vi "Example After.vi"() -> ()   [LabVIEW 2019, in "LSS.lvlib"]
doc: "This example demonstrates how a user can save time developing user interfaces using LSS by showing how a simple application that uses property nodes to change style at runtime can be transitioned to using LSS. The \"Example Before.vi\" contains one way the code could have been written using arrays of property nodes. The \"Example After.vi\" is a functionally equivalent piece of code that uses LSS instead. Example After.vi uses no property nodes or manually created references to perform the exact same operations."
uses:
  LSS.lvlib
  SubVIs/Example SubVIs/Before SubVIs/Themes.ctl
panel:
  in  "CUSTOM":bool
  out "mode":T1
  in  "DIALOG":bool
  in  "NORMAL":bool
  in  "SMALL":bool
  in  "Slide 2":dbl(slide) scale=0.0..10.0
  out "Stat2":dbl
  out "Stat1":dbl
  out "Pressure":dbl
  out "Time":dbl
  in  "Slide":dbl(slide) scale=0.0..10.0
  in  "THEME2":bool
  in  "THEME1":bool
  in  "COMPANY":bool
  in  "SPACE":bool
  out "Mars":picture
  out "Map":picture
  out "SLS":picture
  out "Chart3":dbl(graph)
  out "Chart2":dbl(graph)
  out "Chart1":dbl(graph)
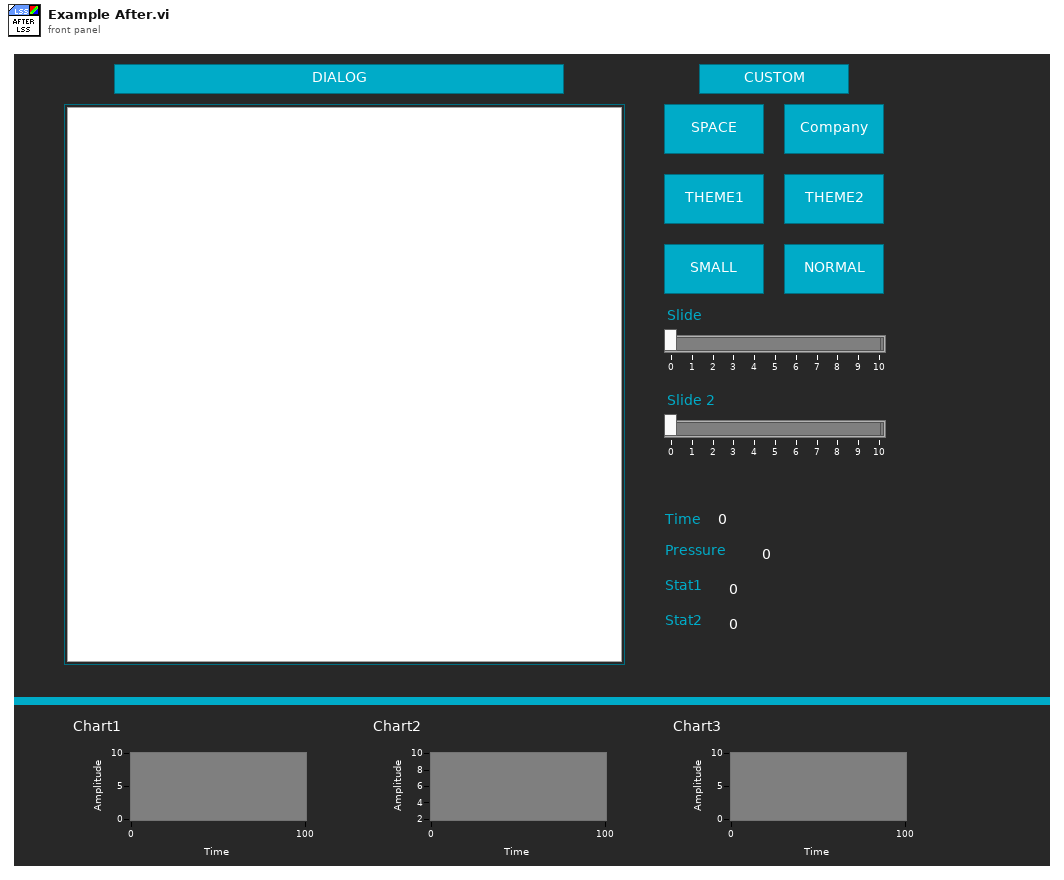
[diagram p1: front panel]
types:
  T1 = typedef "LSS.lvlib/Themes.ctl" = enum16{"SPACE", "COMPANY", "THEME1", "THEME2"}
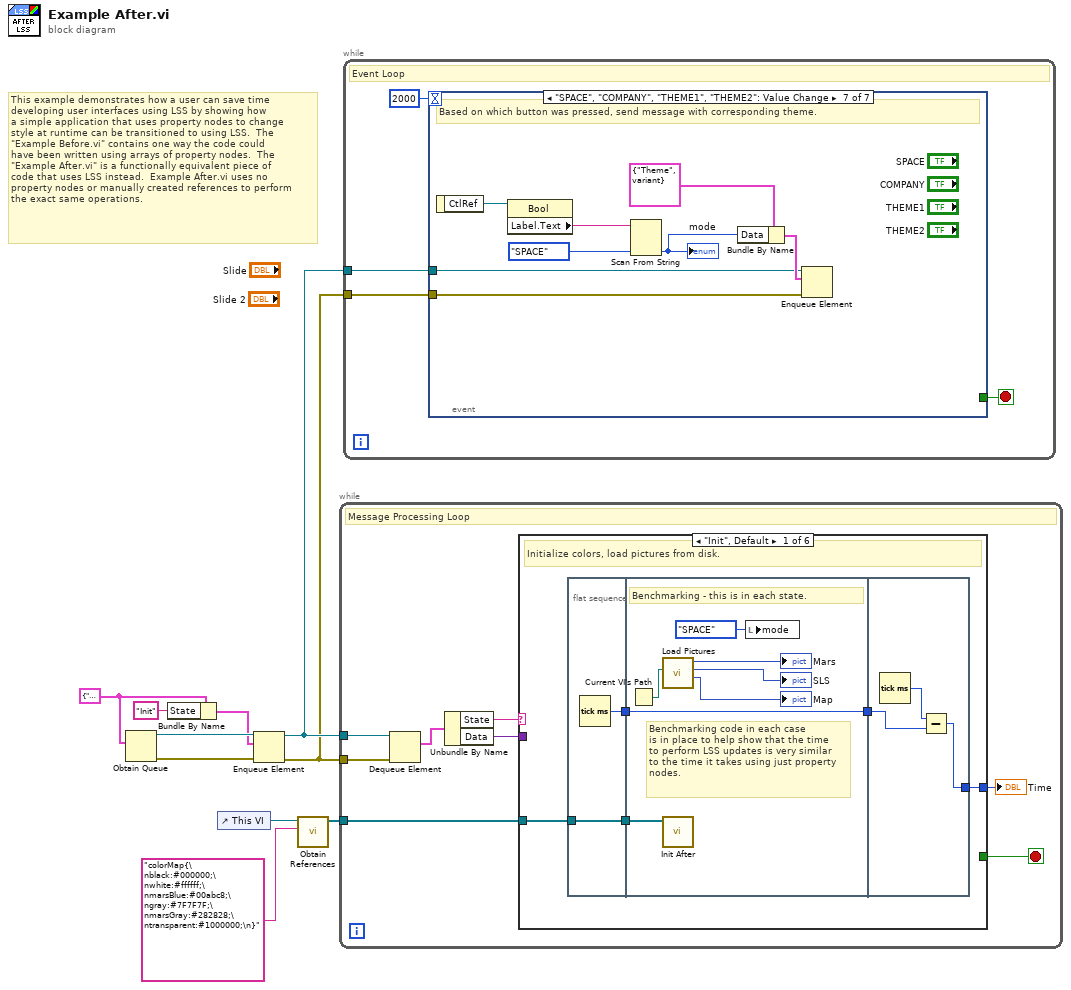
[diagram p0: block diagram]
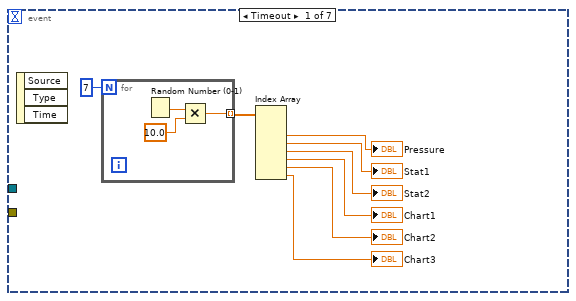
[diagram p2: hidden frame]
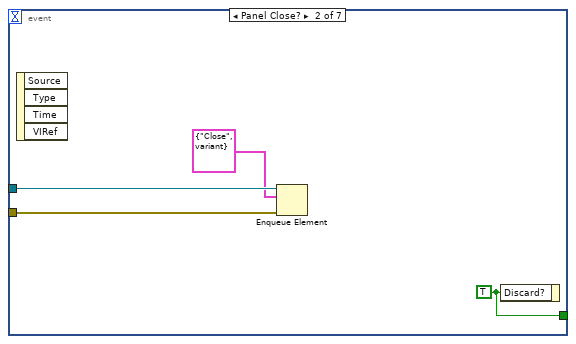
[diagram p3: hidden frame]
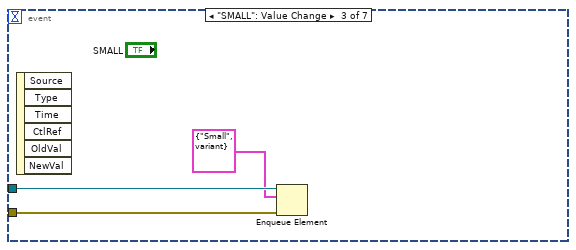
[diagram p4: hidden frame]
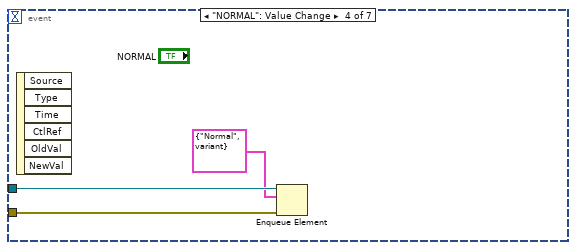
[diagram p5: hidden frame]
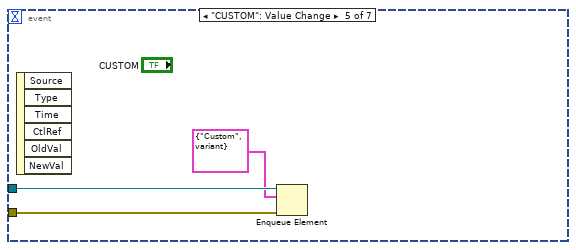
[diagram p6: hidden frame]
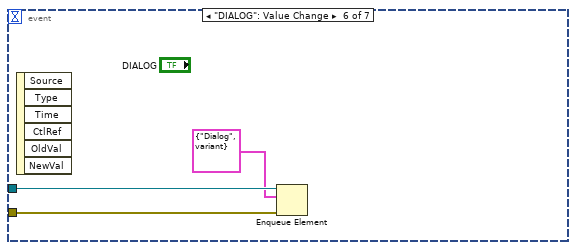
[diagram p7: hidden frame]
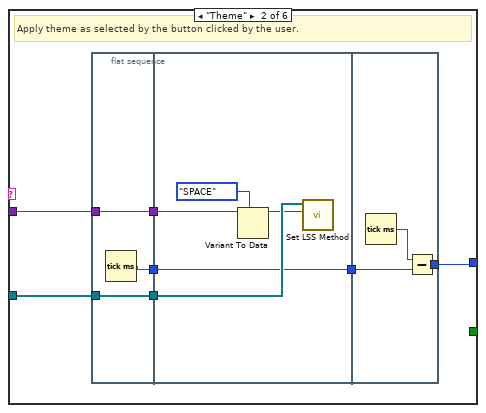
[diagram p8: hidden frame]
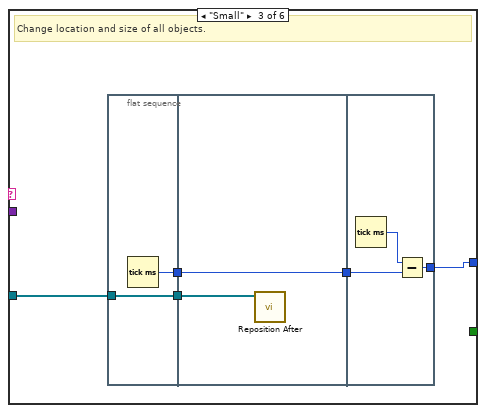
[diagram p9: hidden frame]
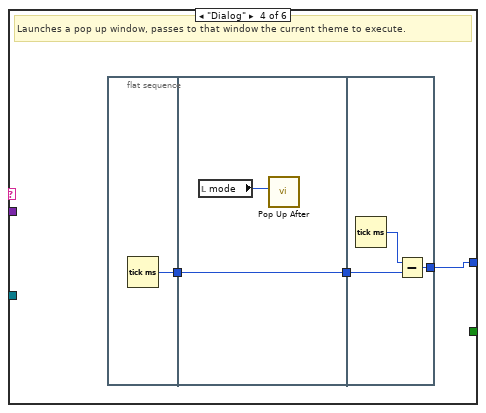
[diagram p10: hidden frame]
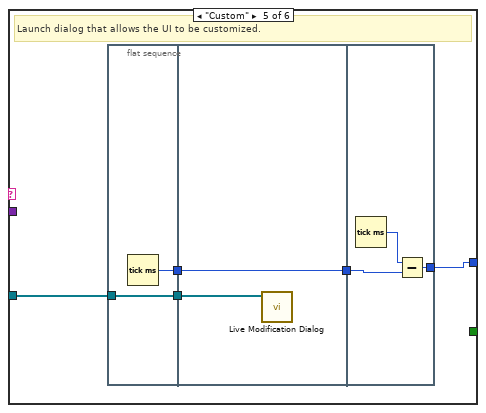
[diagram p11: hidden frame]
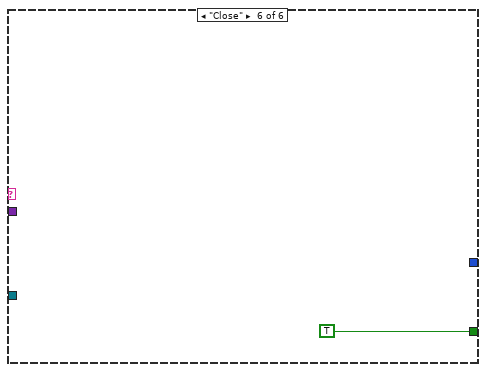
[diagram p12: hidden frame]
diagram:
  w8 = cluster{"State":string, "Data":variant} {"State"="", "Data"=variant}
  # "This example demonstrates how a user can save time\ndeveloping user interfaces using LSS by showing how\na simple application that uses property nodes to change\nstyle at runtime can be transitioned to using LSS.  The\n\"Example Before.vi\" contains one way the code could\nhave been written using arrays of property nodes.  The\n\"Example After.vi\" is a functionally equivalent piece of\ncode that uses LSS instead.  Example After.vi uses no\nproperty nodes or manually created references to perform\nthe exact same operations."
  n1 = Obtain Queue(element data type=w8) -> (queue out=w10:refnum<queue>, error out=w9:errorcluster)  [unwired: 4 in, 1 out]
  n2 = Bundle By Name(cluster=w8, "State"="Init") -> (w6:cluster{"State":string, "Data":variant})
  n3 = control-ref of="This VI"() -> (w3:refnum<vi>)
  n4 = Enqueue Element(queue=w10, element=w6, error in (no error)=w9) -> (queue out=w5:refnum<queue>, error out=w4:errorcluster)  [unwired: 1 in, 1 out]
  n5 = call "Obtain References.vi"("colorMap"="colorMap{\nblack:#000000;\nwhite:#ffffff;\nmarsBlue:#00abc8;\ngray:#7F7F7F;\nmarsGray:#282828;\ntransparent:#1000000;\n}", "VI in"=w3) -> ("Front Panel Objects"=w2:refnum<vi>[])  [unwired: 8 in, 1 out]
  n6 = while {
    tunnel: w5 -> [w18]
    tunnel: w4 -> [w17]
    tunnel: w2 -> [w12]
    stop <- w13 stop-if-true
    # "Message Processing Loop"
    n7 = Dequeue Element(queue=w18, error in (no error)=w17) -> (element=w16:cluster{"State":string, "Data":variant})  [unwired: 1 in, 3 out]
    n8 = Unbundle By Name(w16) -> ("State"=w15:string, "Data"=w14:variant)
    n9 = case shown="\"Init\", Default" w15 {
      tunnel: w14 -> [_ w42 _ _ _ _]
      tunnel: [_ _ _ _ _ TRUE] -> w13
      tunnel: w12 -> [w23 w41 w58 _ w79 _]
      tunnel: [w19 w36 w54 w66 w75 _] -> w11
      frame "Init", Default {
        # "Initialize colors, load pictures from disk."
        n10 = flat-sequence {
          tunnel: w23 -> [w25]
          tunnel: [w25] -> w22
          tunnel: [w24] -> w20
          tunnel: w22 -> [w32]
          tunnel: [w28] -> w21
          tunnel: w20 -> [w28]
          tunnel: w21 -> [w34]
          tunnel: [w33] -> w19
          frame #0 {
            n11 = Tick Count (ms)() -> (millisecond timer value=w24:u32)
          }
          frame #1 {
            # "Benchmarking code in each case\nis in place to help show that the time\nto perform LSS updates is very similar\nto the time it takes using just property\nnodes."
            # "Benchmarking - this is in each state."
            n12 = Current VI's Path() -> (path=w26:path)
            n13 = call "Load Pictures.vi"("Application Directory"=w26) -> ("Map"=→"Map":picture, "Vortex"=→"SLS":picture, "Mars"=→"Mars":picture)  [unwired: 8 in]
            n14 = call "Init After.vi"("UI References"=w32) -> ()  [unwired: 11 in]
            n15 = local write "mode"(Themes."SPACE" ("mode")) -> ()
          }
          frame #2 {
            n16 = Tick Count (ms)() -> (millisecond timer value=w35:u32)
            n17 = Subtract(x=w35, y=w34) -> (x-y=w33:u32)
          }
        }
      }
      frame "Theme" {
        # "Apply theme as selected by the button clicked by the user."
        n18 = flat-sequence {
          tunnel: w41 -> [w44]
          tunnel: w42 -> [w45]
          tunnel: [w45] -> w40
          tunnel: [w44] -> w39
          tunnel: [w43] -> w37
          tunnel: w40 -> [w49]
          tunnel: w39 -> [w48]
          tunnel: [w46] -> w38
          tunnel: w37 -> [w46]
          tunnel: w38 -> [w52]
          tunnel: [w51] -> w36
          frame #0 {
            n19 = Tick Count (ms)() -> (millisecond timer value=w43:u32)
          }
          frame #1 {
            n20 = Variant To Data(type=Themes."SPACE" ("Theme Choice"), Variant=w49) -> (data=w47:T1)  [unwired: 1 in, 1 out]
            n21 = call "Set LSS Method.vi"("Theme Choice"=w47, "Front Panel Objects"=w48) -> ()  [unwired: 10 in]
          }
          frame #2 {
            n22 = Tick Count (ms)() -> (millisecond timer value=w53:u32)
            n23 = Subtract(x=w53, y=w52) -> (x-y=w51:u32)
          }
        }
      }
      frame "Small" {
        # "Change location and size of all objects."
        n24 = flat-sequence {
          tunnel: w58 -> [w60]
          tunnel: [w60] -> w57
          tunnel: [w59] -> w55
          tunnel: w57 -> [w62]
          tunnel: [w61] -> w56
          tunnel: w55 -> [w61]
          tunnel: w56 -> [w64]
          tunnel: [w63] -> w54
          frame #0 {
            n25 = Tick Count (ms)() -> (millisecond timer value=w59:u32)
          }
          frame #1 {
            n26 = call "Reposition After.vi"("Front Panel Objects"=w62) -> ()  [unwired: 11 in]
          }
          frame #2 {
            n27 = Tick Count (ms)() -> (millisecond timer value=w65:u32)
            n28 = Subtract(x=w65, y=w64) -> (x-y=w63:u32)
          }
        }
      }
      frame "Dialog" {
        # "Launches a pop up window, passes to that window the current theme to execute."
        n29 = flat-sequence {
          tunnel: [w69] -> w67
          tunnel: [w71] -> w68
          tunnel: w67 -> [w71]
          tunnel: w68 -> [w73]
          tunnel: [w72] -> w66
          frame #0 {
            n30 = Tick Count (ms)() -> (millisecond timer value=w69:u32)
          }
          frame #1 {
            n31 = local read "mode"() -> (w70:T1)
            n32 = call "Pop Up After.vi"("mode"=w70) -> ()  [unwired: 11 in]
          }
          frame #2 {
            n33 = Tick Count (ms)() -> (millisecond timer value=w74:u32)
            n34 = Subtract(x=w74, y=w73) -> (x-y=w72:u32)
          }
        }
      }
      frame "Custom" {
        # "Launch dialog that allows the UI to be customized."
        n35 = flat-sequence {
          tunnel: w79 -> [w81]
          tunnel: [w81] -> w78
          tunnel: [w80] -> w76
          tunnel: w78 -> [w82]
          tunnel: [w83] -> w77
          tunnel: w76 -> [w83]
          tunnel: w77 -> [w85]
          tunnel: [w84] -> w75
          frame #0 {
            n36 = Tick Count (ms)() -> (millisecond timer value=w80:u32)
          }
          frame #1 {
            n37 = call "Live Modification Dialog.vi"("Front Panel Objects"=w82) -> ()  [unwired: 11 in]
          }
          frame #2 {
            n38 = Tick Count (ms)() -> (millisecond timer value=w86:u32)
            n39 = Subtract(x=w86, y=w85) -> (x-y=w84:u32)
          }
        }
      }
      frame "Close" {
      }
    }
    "Time" <- w11
  }
  n40 = while {
    tunnel: w5 -> [w91]
    tunnel: w4 -> [w90]
    stop <- w89 stop-if-true
    # "Event Loop"
    n41 = event shown="[6] \"SPACE\", \"COMPANY\", \"THEME1\", \"THEME2\": Value Change" {
      selector: _ -> [_ _ _ _ _ _ _]
      dyn-events: _ -> [_ _ _ _ _ _ _]
      timeout: 2000 -> [_ _ _ _ _ _ _]
      tunnel: w91 -> [_ w105 w109 w112 w115 w118 w120]
      tunnel: w90 -> [_ w104 w108 w111 w114 w117 w119]
      tunnel: [_ w106 _ _ _ _ _] -> w89
      event Timeout {
        n42 = event-data() -> ()  [unwired: 1 in, 3 out]
        n43 = for {
          N: 7 -> [_]
          tunnel: [w100] -> w99 mode=indexing
          n44 = Random Number (0-1)() -> (number: 0 to 1=w102:dbl)
          n45 = Multiply(x=w102, y=10.0) -> (x*y=w100:dbl)
        }
        n46 = Index Array(array=w99) -> (element #2=→"Pressure":dbl, element #3=→"Stat1":dbl, element #4=→"Stat2":dbl, element #5=→"Chart1":dbl, element #6=→"Chart2":dbl, element #7=→"Chart3":dbl)  [unwired: 7 in, 1 out]
      }
      event Panel Close? {
        w106 = TRUE ("Discard?")
        n47 = event-data() -> ()  [unwired: 1 in, 4 out]
        n48 = Enqueue Element(queue=w105, element=cluster{"State":string, "Data":variant} {"State"="Close", "Data"=variant}, error in (no error)=w104) -> ()  [unwired: 1 in, 3 out]
        n49 = event-data("Discard?"=w106) -> ()  [unwired: 1 in, 1 out]
      }
      event "SMALL": Value Change {
        n50 = event-data() -> ()  [unwired: 1 in, 6 out]
        n51 = Enqueue Element(queue=w109, element=cluster{"State":string, "Data":variant} {"State"="Small", "Data"=variant}, error in (no error)=w108) -> ()  [unwired: 1 in, 3 out]
      }
      event "NORMAL": Value Change {
        n52 = event-data() -> ()  [unwired: 1 in, 6 out]
        n53 = Enqueue Element(queue=w112, element=cluster{"State":string, "Data":variant} {"State"="Normal", "Data"=variant}, error in (no error)=w111) -> ()  [unwired: 1 in, 3 out]
      }
      event "CUSTOM": Value Change {
        n54 = event-data() -> ()  [unwired: 1 in, 6 out]
        n55 = Enqueue Element(queue=w115, element=cluster{"State":string, "Data":variant} {"State"="Custom", "Data"=variant}, error in (no error)=w114) -> ()  [unwired: 1 in, 3 out]
      }
      event "DIALOG": Value Change {
        n56 = event-data() -> ()  [unwired: 1 in, 6 out]
        n57 = Enqueue Element(queue=w118, element=cluster{"State":string, "Data":variant} {"State"="Dialog", "Data"=variant}, error in (no error)=w117) -> ()  [unwired: 1 in, 3 out]
      }
      event "SPACE", "COMPANY", "THEME1", "THEME2": Value Change {
        # "Based on which button was pressed, send message with corresponding theme."
        n58 = event-data() -> ("CtlRef"=w121:refnum<vi>)  [unwired: 1 in]
        n59 = property class="Bool"(reference=w121) -> ("Label.Text"=w124:string)  [unwired: 1 in, 2 out]
        n60 = Scan From String(input string=w124, default 1=Themes."SPACE" ("Theme Choice")) -> (output 1=w125:T1)  [unwired: 3 in, 3 out]
        "mode" <- w125
        n61 = Bundle By Name(cluster=cluster{"State":string, "Data":variant} {"State"="Theme", "Data"=variant} ("element"), "Data"=w125) -> (w123:cluster{"State":string, "Data":variant})
        n62 = Enqueue Element(queue=w120, element=w123, error in (no error)=w119) -> ()  [unwired: 1 in, 3 out]
      }
    }
  }
